vi "Update Serial Number1.vi"(8 "error in":errorcluster, 11 "Result":enum16{"Pass", "Fail"}(ring)) -> (0 "error out":errorcluster, 1 "Serial Number":dbl, 3 "Serial number":string)   [LabVIEW 2024]
uses:
  C:/Users/enProducts/Downloads/KIA_Enproducts/KIA_Enproducts/Global VIs/Controls/Read Write.ctl
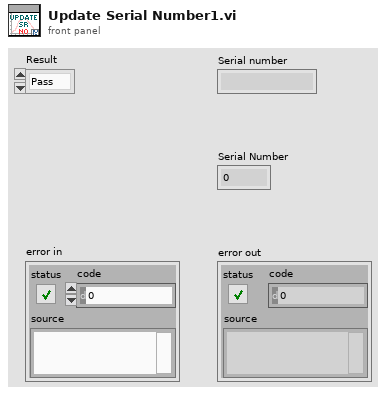
[diagram p1: front panel]
types:
  T1 = typedef "SERIAL N0.ctl" = string
  T2 = typedef "Read Write.ctl" = enum16{"Read", "Write"}
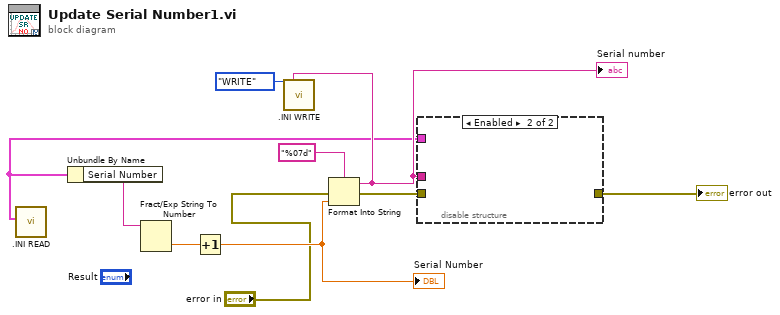
[diagram p0: block diagram]
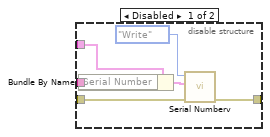
[diagram p2: hidden frame]
diagram:
  n1 = call ".INI READ.vi"() -> ("Serail No"=w3:cluster{"Serial Number":T1})  [unwired: 4 in, 7 out]
  n2 = Unbundle By Name(w3) -> ("Serial Number"=w6:T1)
  n3 = Fract/Exp String To Number(string=w6) -> (number=w5:dbl)  [unwired: 3 in, 1 out]
  n4 = Increment(x=w5) -> (x+1=w4:dbl)
  "Serial Number" <- w4
  n5 = Format Into String(format string="%07d", error in="error in", w4) -> (resulting string=w10:string, error out=w8:errorcluster)  [unwired: 1 in]
  "Serial number" <- w10
  n6 = call ".INI WRITE.vi"("Enum"=enum16{"READ", "WRITE"}."WRITE", "Serial Number"=w10) -> ()  [unwired: 26 in]
  n7 = disable-structure shown="Enabled" {
    disable-tunnel: w10 -> [w16 _]
    disable-tunnel: w3 -> [w13 _]
    disable-tunnel: w8 -> [w12 _]
    disable-tunnel: [w11 _] -> w7
    frame Disabled {
      n8 = Bundle By Name(cluster=w13, "Serial Number"=w16) -> (w14:cluster{"Serial Number":T1})
      n9 = call "Serial Numberv.vi"("error in"=w12, "Serial No"=w14, "Read Write"=Read_Write."Write") -> ("error out"=w11:errorcluster)  [unwired: 7 in, 1 out]
    }
    frame Enabled {
    }
  }
  "error out" <- w7
